vi "test - NESTED Write with the section name you write.vi"(8 "error in (no error)":errorcluster, 11 "TestCase in":refnum<class "csm-ini-variable-addon.lvclass">) -> (0 "error out":errorcluster, 3 "TestCase out":refnum<class "csm-ini-variable-addon.lvclass">)   [LabVIEW 2017, in "csm-ini-variable-addon.lvclass"]
uses:
  csm-ini-variable-addon.lvclass
  INI-Static-Variable-Support/INI-Static-Variable-Support.lvlib
  a890fef7-7f1d-42c9-b9db-12bb2b441289.vi
  25df91f5-a8e9-4b30-a15a-ad417606420d.vi
  4506128f-911b-4b09-9ad5-a28d51cf287f.vi
  fd1f1403-f650-4147-a5d0-7fa8994ff20a.vi
panel:
  # "Connector Pane"
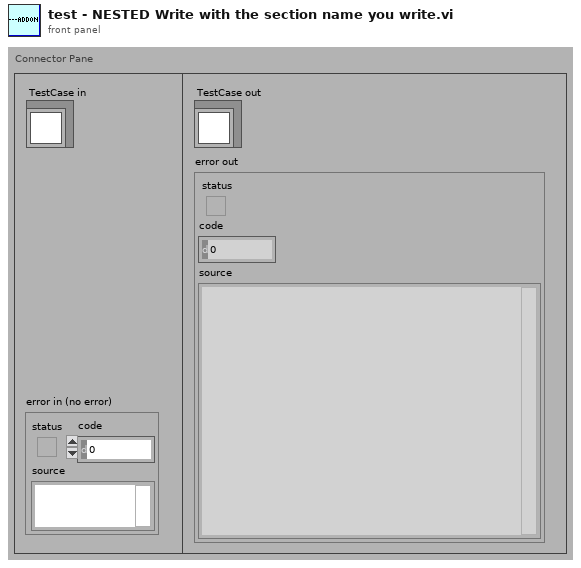
[diagram p1: front panel]
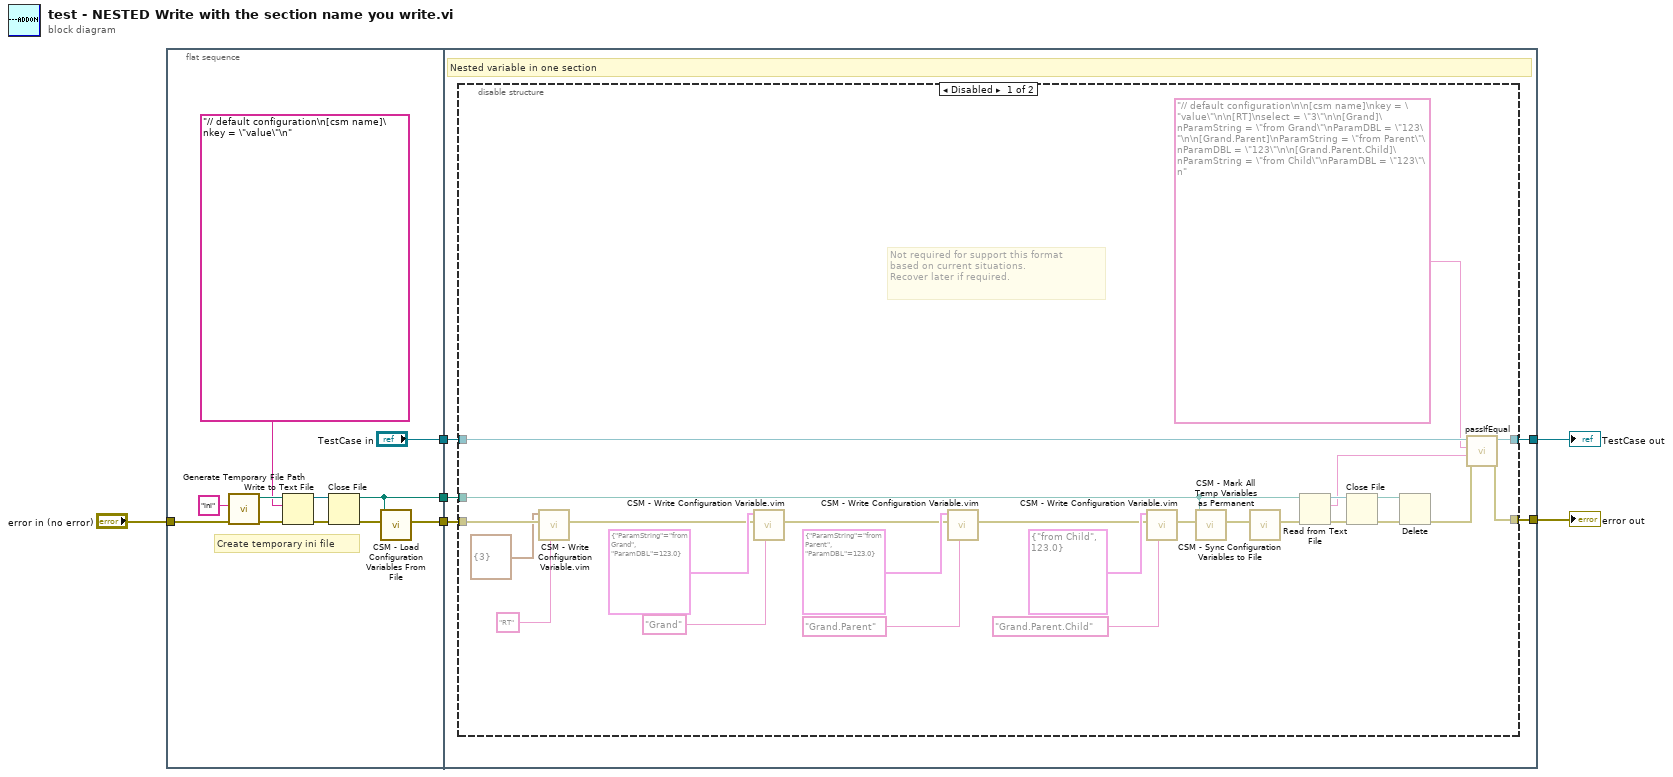
[diagram p0: block diagram]
diagram:
  n1 = flat-sequence {
    tunnel: "error in (no error)" -> [w10]
    tunnel: [w8] -> w5
    tunnel: ["TestCase in"] -> w4
    tunnel: [w7] -> w1
    tunnel: w5 -> [w19]
    tunnel: w4 -> [w18]
    tunnel: [w22] -> w3
    tunnel: [w21] -> w2
    tunnel: w1 -> [w20]
    frame #0 {
      # "Create temporary ini file"
      n2 = call <vilib>:"Generate Temporary File Path.vi"("error in (no error)"=w10, "Temporary File Extension (tmp)"="ini") -> ("error out"=w17:errorcluster, "Unique Temporary File Path"=w14:path)  [unwired: 8 in]
      n3 = Write to Text File(file (use dialog)=w14, text="// default configuration\n[csm name]\nkey = \"value\"\n", error in=w17) -> (refnum out=w13:refnum<file>, error out=w15:errorcluster)  [unwired: 1 in, 1 out]
      n4 = Close File(refnum=w13, error in=w15) -> (path=w7:path, error out=w12:errorcluster)
      n5 = call "CSM - Load Configuration Variables From File.vi"("error in (no error)"=w12, "Path"=w7) -> ("error out"=w8:errorcluster)  [unwired: 7 in]
    }
    frame #1 {
      # "Nested variable in one section"
      n6 = disable-structure shown="Disabled" {
        disable-tunnel: [w48 w50] -> w22
        disable-tunnel: [w47 w49] -> w21
        disable-tunnel: w20 -> [w35 _]
        disable-tunnel: w19 -> [w29 w49]
        disable-tunnel: w18 -> [w26 w50]
        frame Disabled {
          # "Not required for support this format\nbased on current situations.\nRecover later if required."
          n7 = call "CSM - Write Configuration Variable.vim"("Section Name(\"\" as Default)"="RT" ("Section Name(\"\" as Default)"), "error in (no error)"=w29, "Variant"=cluster{"select":i32} {"select"=3}) -> ("error out"=w30:errorcluster)  [unwired: 5 in, 1 out]
          n8 = call "CSM - Write Configuration Variable.vim"("Section Name(\"\" as Default)"="Grand" ("Section Name(\"\" as Default)"), "error in (no error)"=w30, "Variant"=cluster{"ParamString":string, "ParamDBL":dbl} {"ParamString"="from Grand", "ParamDBL"=123.0}) -> ("error out"=w42:errorcluster)  [unwired: 5 in, 1 out]
          n9 = call "CSM - Write Configuration Variable.vim"("Section Name(\"\" as Default)"="Grand.Parent" ("Section Name(\"\" as Default)"), "error in (no error)"=w42, "Variant"=cluster{"ParamString":string, "ParamDBL":dbl} {"ParamString"="from Parent", "ParamDBL"=123.0}) -> ("error out"=w39:errorcluster)  [unwired: 5 in, 1 out]
          n10 = call "CSM - Write Configuration Variable.vim"("Section Name(\"\" as Default)"="Grand.Parent.Child" ("Section Name(\"\" as Default)"), "error in (no error)"=w39, "Variant"=cluster{"ParamString":string, "ParamDBL":dbl} {"ParamString"="from Child", "ParamDBL"=123.0}) -> ("error out"=w38:errorcluster)  [unwired: 5 in, 1 out]
          n11 = call "CSM - Mark All Temp Variables as Permanent.vi"("error in (no error)"=w38, "Path(\"\" to use default ini)"=w35) -> ("error out"=w37:errorcluster)  [unwired: 7 in]
          n12 = call "CSM - Sync Configuration Variables to File.vi"("error in (no error)"=w37) -> ("error out"=w36:errorcluster)  [unwired: 8 in]
          n13 = Read from Text File(file (use dialog)=w35, error in=w36) -> (refnum out=w34:refnum<file>, text=w24:string, error out=w33:errorcluster)  [unwired: 2 in, 1 out]
          n14 = Close File(refnum=w34, error in=w33) -> (path=w31:path, error out=w32:errorcluster)
          n15 = Delete(path (use dialog)=w31, error in=w32) -> (error out=w25:errorcluster)  [unwired: 3 in, 2 out]
          n16 = call-dynamic "passIfEqual.vi"("error in (no error)"=w25, "y"=w24, "x"="// default configuration\n\n[csm name]\nkey = \"value\"\n\n[RT]\nselect = \"3\"\n\n[Grand]\nParamString = \"from Grand\"\nParamDBL = \"123\"\n\n[Grand.Parent]\nParamString = \"from Parent\"\nParamDBL = \"123\"\n\n[Grand.Parent.Child]\nParamString = \"from Child\"\nParamDBL = \"123\"\n" ("text"), "TestCase in"=w26) -> ("error out"=w47:errorcluster, "TestCase out"=w48:refnum<class "csm-ini-variable-addon.lvclass">)  [unwired: 6 in]
        }
        frame Enabled {
        }
      }
    }
  }
  "error out" <- w2
  "TestCase out" <- w3
